vi "CloseVIs.vi"() -> (0 "error out":errorcluster)   [LabVIEW 2017]
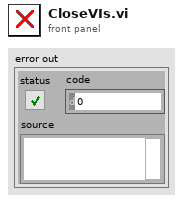
[diagram p1: front panel]
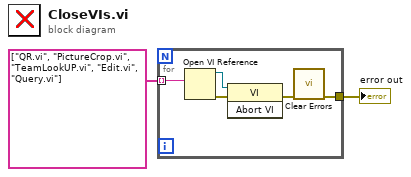
[diagram p0: block diagram]
diagram:
  n1 = for {
    tunnel: [w7] -> w1
    tunnel: string[] ["QR.vi", "PictureCrop.vi", "TeamLookUP.vi", "Edit.vi", "Query.vi"] ("name or relative path") -> [w5] mode=indexing
    n2 = Open VI Reference(vi path=w5) -> (vi reference=w4:refnum<vi>, error out=w3:errorcluster)  [unwired: 5 in]
    n3 = invoke class="VI" method="Abort VI"(reference=w4, error in=w3) -> (error out=w6:errorcluster)  [unwired: 1 in, 2 out]
    n4 = call <vilib>:"Clear Errors.vi"("error in (no error)"=w6) -> ("error out"=w7:errorcluster)  [unwired: 5 in, 1 out]
  }
  "error out" <- w1
